vi "Resize Button to Fit Text.vi"(10 "error in (no error)":errorcluster, 11 "Boolean in":refnum<vi>) -> (2 "error out":errorcluster, 3 "Boolean out":refnum<vi>)   [LabVIEW 2021, in "Buttons.lvlib"]
uses:
  Buttons.lvlib
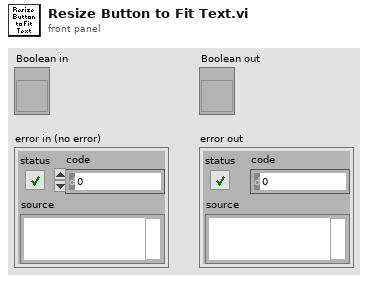
[diagram p1: front panel]
types:
  T1 = cluster{"horizontal":enum16{"left", "center", "right"}, "vertical":enum16{"top", "center", "bottom"}}
  T2 = cluster{"Font Name:":string, "Size":i16, "Strikeout?":bool, "Italic?":bool, "Underline?":bool, "Outline?":bool, "Shadow?":bool, "Bold?":bool}
  T3 = typedef "LVFontTypeDef.ctl" = cluster{"Font Name":string, "Size":u16, "Bold":bool, "Italic":bool, "Underline":bool, "Strikeout":bool, "Color":u32}
  T4 = cluster{"left":i16, "top":i16, "right":i16, "bottom":i16}
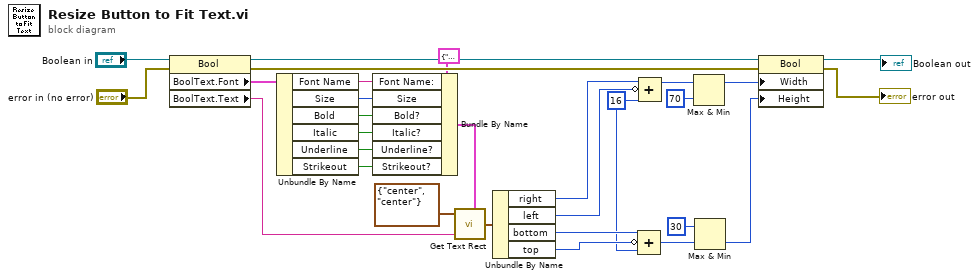
[diagram p0: block diagram]
diagram:
  w6 = u32 16 ("value")
  n1 = property class="Bool"(reference="Boolean in", error in="error in (no error)") -> (reference out=w27:refnum<vi>, error out=w26:errorcluster, "BoolText.Font"=w20:T3, "BoolText.Text"=w22:string)
  n2 = Unbundle By Name(w20) -> ("Font Name"=w19:string, "Size"=w17:u16, "Bold"=w18:bool, "Italic"=w16:bool, "Underline"=w15:bool, "Strikeout"=w14:bool)
  n3 = Bundle By Name(cluster=T2 {"Font Name:"="", "Size"=0, "Strikeout?"=FALSE, "Italic?"=FALSE, "Underline?"=FALSE, "Outline?"=FALSE, "Shadow?"=FALSE, "Bold?"=FALSE} ("[user-specified font]"), "Font Name:"=w19, "Size"=w17, "Bold?"=w18, "Italic?"=w16, "Underline?"=w15, "Strikeout?"=w14) -> (w13:T2)
  n4 = call <vilib>:"Get Text Rect.vi"("alignment(left, top)"=T1 {"horizontal"=enum."center", "vertical"=enum."center"}, "text"=w22, "[user-specified font]"=w13) -> ("rect"=w11:T4)  [unwired: 6 in]
  n5 = Unbundle By Name(w11) -> ("right"=w10:i16, "left"=w9:i16, "bottom"=w8:i16, "top"=w7:i16)
  n6 = Compound Arithmetic op=unknown(w8, invert w7, w6) -> (w5:u32)
  n7 = Compound Arithmetic op=unknown(w10, invert w9, w6) -> (w25:u32)
  n8 = Max & Min(x=w25, y=u32 70) -> (max(x,y)=w4:u32)  [unwired: 1 out]
  n9 = Max & Min(x=u32 30, y=w5) -> (min(x,y)=w2:u32)  [unwired: 1 out]
  n10 = property class="Bool"(reference=w27, error in=w26, "Width"=w4, "Height"=w2) -> (reference out=→"Boolean out":refnum<vi>, error out=→"error out":errorcluster)
